vi "warning calibrazioni.vi"(9 "millennio":i32=2000, 10 "PAGINE TRASDUTTORI":string[][](array[string]), 11 "Table in":refnum<vi>) -> ()   [LabVIEW 2019]
uses:
  <vilib>/Utility/miscctls.llb/LVRowAndColumnTypeDef.ctl
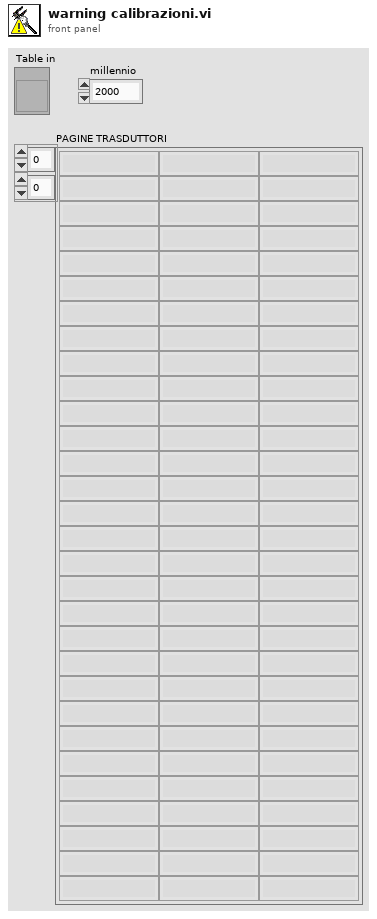
[diagram p1: front panel]
types:
  T1 = typedef "LVRowAndColumnTypeDef.ctl" = cluster{"Row":i32, "Column":i32}
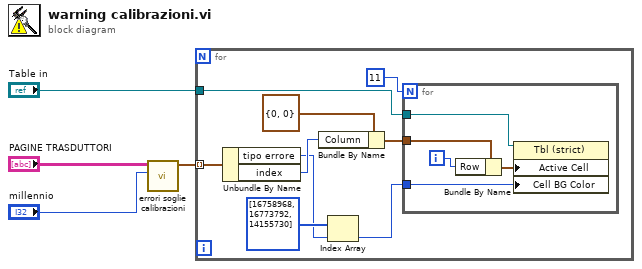
[diagram p0: block diagram]
diagram:
  n1 = call "errori soglie calibrazioni.vi"("millennio"="millennio", "PAGINE TRASDUTTORI"="PAGINE TRASDUTTORI") -> ("Array errori"=w3:cluster{"tipo errore":i32, "index":i32}[])  [unwired: 9 in]
  n2 = for {
    tunnel: w3 -> [w11] mode=indexing
    tunnel: "Table in" -> [w13]
    n3 = Unbundle By Name(w11) -> ("tipo errore"=w6:i32, "index"=w10:i32)
    n4 = Bundle By Name(cluster=T1 {"Row"=0, "Column"=0} ("Active Cell:Active Cell"), "Column"=w10) -> (w9:T1)
    n5 = Index Array(array=u32[] [16758968, 16773792, 14155730], index=w6) -> (element=w5:u32)
    n6 = for {
      N: 11 -> [_]
      tunnel: w13 -> [w18]
      tunnel: w9 -> [w17]
      tunnel: w5 -> [w14]
      i -> [w16]
      n7 = Bundle By Name(cluster=w17, "Row"=w16) -> (w15:T1)
      n8 = property class="Tbl (strict)"(reference=w18, "Active Cell"=w15, "Cell BG Color"=w14) -> ()  [unwired: 1 in, 2 out]
    }
  }
